vi "Configure Alarm Math.vi"(0 "VISA resource name":refnum<visa-resource-name>, 1 "Alarm Type (0 : High limit alarm)":i32(ring) items=["H", "L", "TH", "TL"], 2 "Enable Detect (False)":bool, 3 "Relay Number (0)":i32 min=0 max=1000, 5 "Math Channel (001)":string="001", 7 "Alarm Number (1)":i32=1 min=1 max=4 step=1, 9 "Enable Alarm (False)":bool, 11 "error in (no error)":errorcluster, 12 "Alarm Value (0)":i32 min=-9999999 max=99999999 step=1 format="%#_8g", 13 "Output Type (0: Off)":u16(ring) items=["Off", "DO", "Internal switch"]) -> (4 "VISA resource name out":refnum<visa-resource-name>, 6 "Math Channel":string, 8 "Alarm Number":i32, 15 "error out":errorcluster)   [LabVIEW 2020, in "Yokogawa GX Series.lvlib"]
doc: "Sets the alarm of the mathematical channel.\n\nCommand: SAlarmMath"
uses:
  <instrlib>/Yokogawa GX Series/Yokogawa GX Series.lvlib
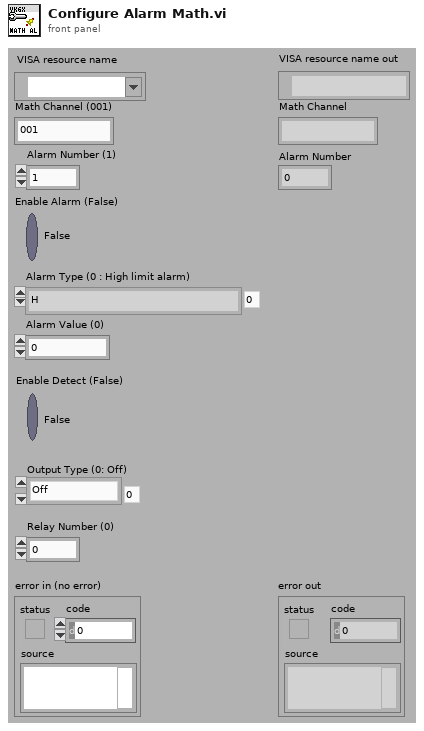
[diagram p1: front panel]
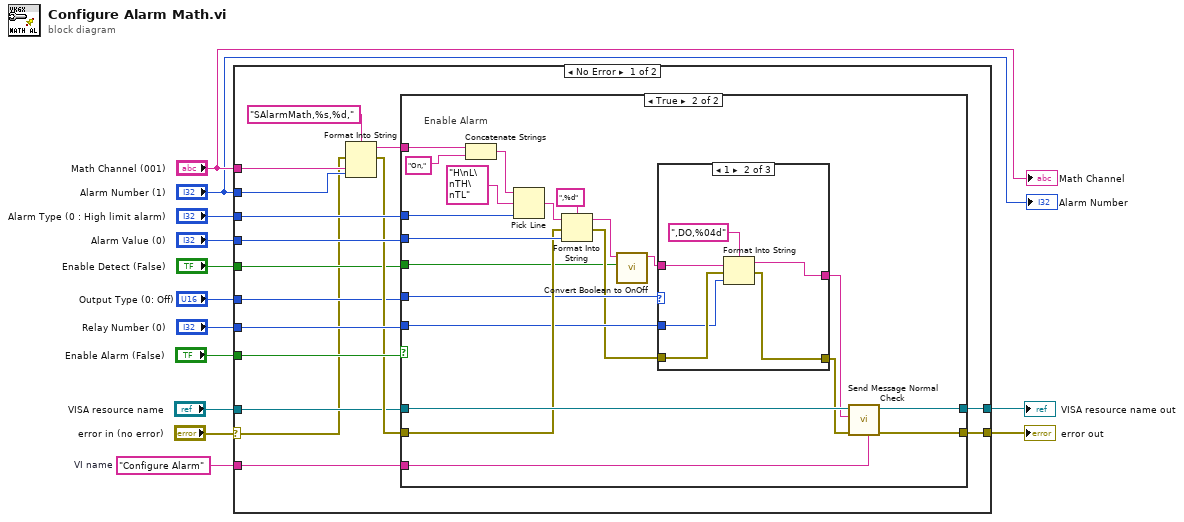
[diagram p0: block diagram]
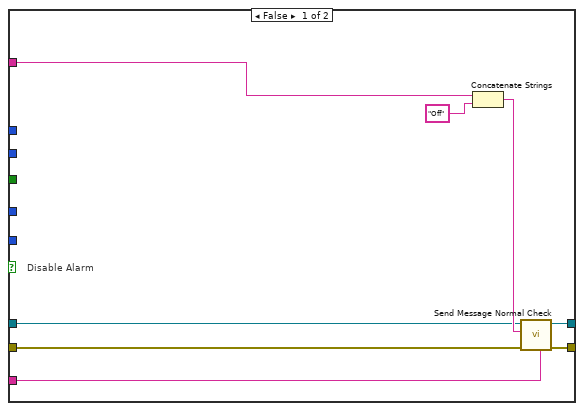
[diagram p2: hidden frame]
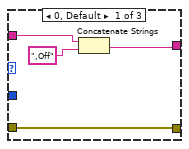
[diagram p3: hidden frame]
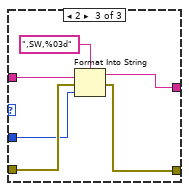
[diagram p4: hidden frame]
diagram:
  w10 = "Configure Alarm"  # VI name
  n1 = case shown="No Error" "error in (no error)" {
    selector: "error in (no error)" -> [w14 w75]
    tunnel: "Enable Alarm (False)" -> [w28 _]
    tunnel: "Alarm Type (0 : High limit alarm)" -> [w26 _]
    tunnel: "Alarm Value (0)" -> [w25 _]
    tunnel: w10 -> [w24 _]
    tunnel: [w23 w76] -> w9
    tunnel: "Relay Number (0)" -> [w22 _]
    tunnel: "Output Type (0: Off)" -> [w20 _]
    tunnel: "Enable Detect (False)" -> [w19 _]
    tunnel: "VISA resource name" -> [w18 w76]
    tunnel: "Math Channel (001)" -> [w17 _]
    tunnel: "Alarm Number (1)" -> [w16 _]
    tunnel: [w15 w75] -> w2
    frame No Error {
      n2 = Format Into String(format string="SAlarmMath,%s,%d,", error in=w14, w17, w16) -> (resulting string=w27:string, error out=w21:errorcluster)  [unwired: 1 in]
      n3 = case shown="True" w28 {
        tunnel: w27 -> [w36 w56]
        tunnel: w26 -> [_ w57]
        tunnel: w25 -> [_ w53]
        tunnel: w18 -> [w34 w49]
        tunnel: w24 -> [w33 w52]
        tunnel: [w32 w42] -> w23
        tunnel: [w31 w41] -> w15
        tunnel: w22 -> [_ w45]
        tunnel: w21 -> [w30 w48]
        tunnel: w20 -> [_ w47]
        tunnel: w19 -> [_ w38]
        frame False {
          # "Disable Alarm"
          n4 = Concatenate Strings(w36, "Off") -> (w35:string)
          n5 = call <instrlib>:"Send Message Normal Check.vi"("Source (\"\")"=w33, "error in (no error)"=w30, "Send Message (\"\")"=w35, "VISA resource name"=w34) -> ("error out"=w31:errorcluster, "VISA resource name out"=w32:refnum<visa-resource-name>)  [unwired: 2 in, 4 out]
        }
        frame True {
          # "Enable Alarm"
          n6 = Concatenate Strings(w56, "On,") -> (w50:string)
          n7 = Pick Line(string ("")=w50, multi-line string="H\nL\nTH\nTL", line index=w57) -> (output string=w54:string)
          n8 = Format Into String(format string=",%d", initial string=w54, error in=w48, w53) -> (resulting string=w39:string, error out=w44:errorcluster)
          n9 = call <instrlib>:"Convert Boolean to OnOff.vi"("On/Off"=w38, "Initial String (\"\")"=w39) -> ("Resulting String"=w40:string)  [unwired: 9 in]
          n10 = case shown="1" w47 {
            tunnel: w40 -> [w62 w68 w74]
            tunnel: [w60 w65 w71] -> w46
            tunnel: w45 -> [_ w63 w69]
            tunnel: w44 -> [w59 w67 w73]
            tunnel: [w59 w64 w70] -> w43
            frame 0, Default {
              n11 = Concatenate Strings(w62, ",Off") -> (w60:string)
            }
            frame 1 {
              n12 = Format Into String(format string=",DO,%04d", initial string=w68, error in=w67, w63) -> (resulting string=w65:string, error out=w64:errorcluster)
            }
            frame 2 {
              n13 = Format Into String(format string=",SW,%03d", initial string=w74, error in=w73, w69) -> (resulting string=w71:string, error out=w70:errorcluster)
            }
          }
          n14 = call <instrlib>:"Send Message Normal Check.vi"("Source (\"\")"=w52, "error in (no error)"=w43, "Send Message (\"\")"=w46, "VISA resource name"=w49) -> ("error out"=w41:errorcluster, "VISA resource name out"=w42:refnum<visa-resource-name>)  [unwired: 2 in, 4 out]
        }
      }
    }
    frame Error {
    }
  }
  "error out" <- w2
  "VISA resource name out" <- w9
  "Math Channel" <- "Math Channel (001)"
  "Alarm Number" <- "Alarm Number (1)"
